vi "CPU temperature.vi"(9 "error in (no error)":errorcluster) -> (1 "error out":errorcluster, 2 "average CPU temp (ºC)":dbl, 4 "# temp sensors":u8)   [LabVIEW 2020]
doc: "Retrieves average CPU temp, if available. No warranty, use it at your own risk.\n\n© Aitor Solar, 2019.\nContact: aitor.solar@gmail.com"
uses:
  C:/Users/Josh/Desktop/code/sandbox/ni/read_temp/OpenHardwareMonitorLib.dll
  OpenHardwareMonitorLib.dll
  <vilib>/Analysis/baseanly.llb/Mean (DBL).vi
  <vilib>/Analysis/NI_AALBase.lvlib
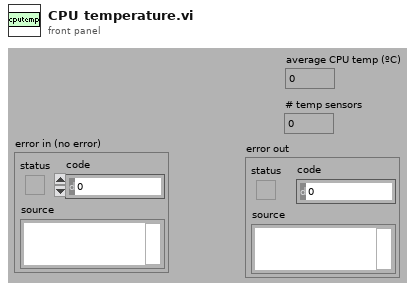
[diagram p1: front panel]
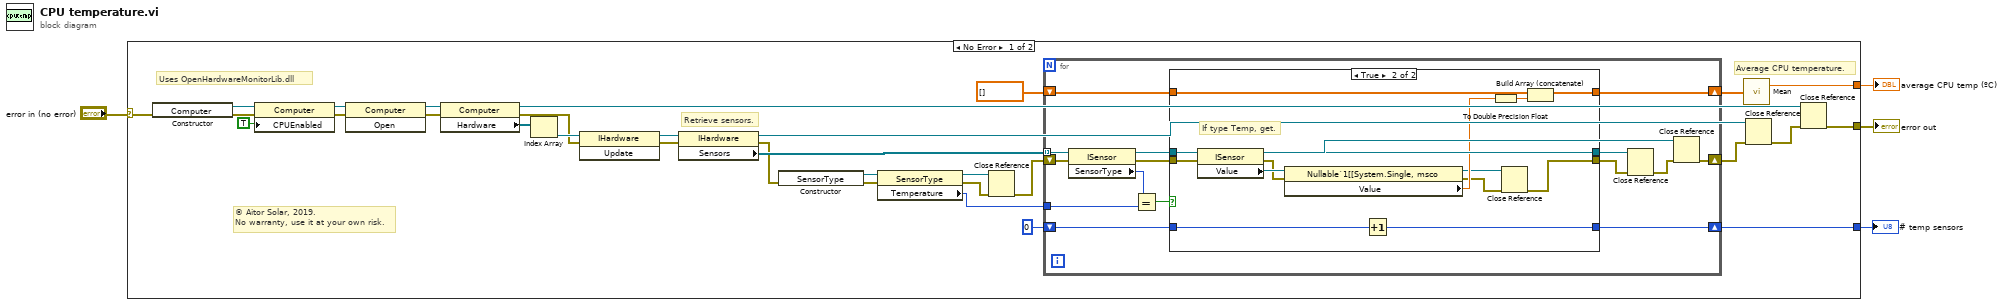
[diagram p0: block diagram]
diagram:
  n1 = case shown="No Error" "error in (no error)" {
    selector: "error in (no error)" -> [w16 w69]
    tunnel: [w22 _] -> w4
    tunnel: [w17 w69] -> w3
    tunnel: [w6 _] -> w1
    frame No Error {
      # "© Aitor Solar, 2019.\nNo warranty, use it at your own risk."
      # "Uses OpenHardwareMonitorLib.dll"
      # "Average CPU temperature."
      # "Retrieve sensors."
      n2 = constructor class="Computer"(error in=w16) -> (reference out=w10:refnum<k24>, error out=w15:errorcluster)  [unwired: 2 in, 1 out]
      n3 = property class="Computer"(reference=w10, error in=w15, "CPUEnabled"=TRUE) -> (reference out=w11:refnum<k24>, error out=w14:errorcluster)
      n4 = invoke class="Computer" method="Open"(reference=w11, error in=w14) -> (reference out=w12:refnum<k24>, error out=w13:errorcluster)  [unwired: 1 in, 1 out]
      n5 = property class="Computer"(reference=w12, error in=w13) -> (reference out=w18:refnum<k24>, error out=w30:errorcluster, "Hardware"=w35:refnum<k24>[])
      n6 = Index Array(array=w35) -> (element=w32:refnum<k24>)  [unwired: 1 in]
      n7 = invoke class="IHardware" method="Update"(reference=w32, error in=w30) -> (reference out=w31:refnum<k24>, error out=w29:errorcluster)  [unwired: 1 in, 1 out]
      n8 = property class="IHardware"(reference=w31, error in=w29) -> (reference out=w20:refnum<k24>, error out=w26:errorcluster, "Sensors"=w33:refnum<k24>[])
      n9 = constructor class="SensorType"(error in=w26) -> (reference out=w27:refnum<k24>, error out=w28:errorcluster)  [unwired: 2 in, 1 out]
      n10 = property class="SensorType"(reference=w27, error in=w28) -> (reference out=w21:refnum<k24>, error out=w8:errorcluster, "Temperature"=w25:i32)
      n11 = Close Reference(reference=w21, error in (no error)=w8) -> (error out=w7:errorcluster)
      n12 = for {
        tunnel: w33 -> [w49] mode=indexing
        shift-right: [w41] -> w9
        shift-left: w7 -> [w48]
        tunnel: w25 -> [w46]
        shift-right: [w50] -> w23
        shift-left: dbl[] [] -> [w44]
        shift-right: [w37] -> w6
        shift-left: u8 0 -> [w36]
        n13 = property class="ISensor"(reference=w49, error in=w48) -> (reference out=w38:refnum<k24>, error out=w47:errorcluster, "SensorType"=w39:i32)
        n14 = Equal?(x=w39, y=w46) -> (x = y?=w45:bool)
        n15 = case shown="True" w45 {
          tunnel: [w54 w67] -> w50
          tunnel: w47 -> [w53 w65]
          tunnel: w44 -> [w54 w68]
          tunnel: [w53 w58] -> w43
          tunnel: [w52 w63] -> w42
          tunnel: w38 -> [w52 w64]
          tunnel: [w51 w56] -> w37
          tunnel: w36 -> [w51 w55]
          frame False {
          }
          frame True {
            # "If type Temp, get."
            n16 = property class="ISensor"(reference=w64, error in=w65) -> (reference out=w63:refnum<k24>, error out=w57:errorcluster, "Value"=w62:refnum<k24>)
            n17 = property class="Nullable`1[[System.Single, msco"(reference=w62, error in=w57) -> (reference out=w60:refnum<k24>, error out=w59:errorcluster, "Value"=w61:sgl)
            n18 = Increment(x=w55) -> (x+1=w56:u8)
            n19 = To Double Precision Float(number=w61) -> (double precision float=w66:dbl)
            n20 = Close Reference(reference=w60, error in (no error)=w59) -> (error out=w58:errorcluster)
            n21 = Build Array (concatenate)(w68, w66) -> (w67:dbl[])
          }
        }
        n22 = Close Reference(reference=w42, error in (no error)=w43) -> (error out=w40:errorcluster)
        n23 = Close Reference(reference=w38, error in (no error)=w40) -> (error out=w41:errorcluster)
      }
      n24 = call-poly <vilib>:"Mean.vi"("X"=w23) -> ("mean"=w22:dbl)  [unwired: 1 out]
      n25 = Close Reference(reference=w20, error in (no error)=w9) -> (error out=w19:errorcluster)
      n26 = Close Reference(reference=w18, error in (no error)=w19) -> (error out=w17:errorcluster)
    }
    frame Error {
    }
  }
  "average CPU temp (ºC)" <- w4
  "error out" <- w3
  "# temp sensors" <- w1
